vi "DataToVariant.vi"(1 "Data":string[][](table)) -> (0 "Variant":variant)   [LabVIEW 2014]
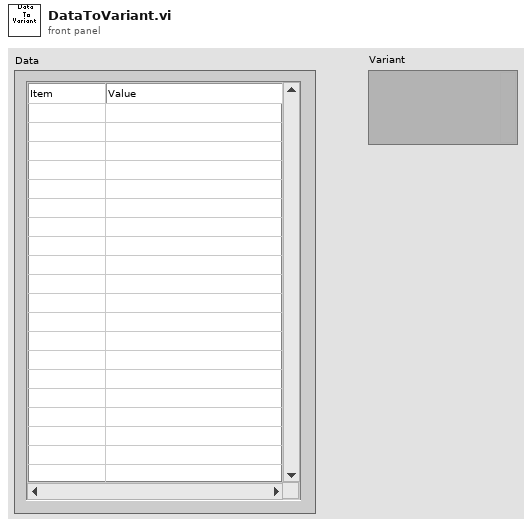
[diagram p1: front panel]
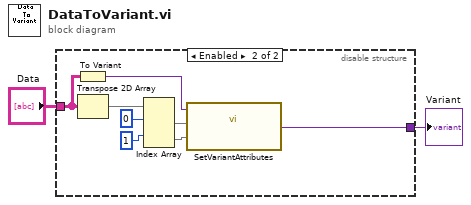
[diagram p0: block diagram]
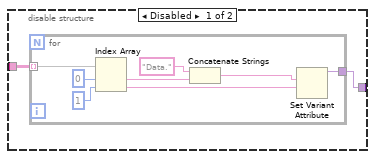
[diagram p2: hidden frame]
diagram:
  n1 = disable-structure shown="Enabled" {
    disable-tunnel: "Data" -> [w4 w20]
    disable-tunnel: [w3 w13] -> w1
    frame Disabled {
      n2 = for {
        tunnel: w4 -> [w12] mode=indexing
        tunnel: [w8] -> w3
        n3 = Index Array(array=w12, index #1=0 ("index"), index #2=1 ("index")) -> (element #1=w6:string, element #2=w9:string)
        n4 = Concatenate Strings("Data." ("string"), w6) -> (w5:string)
        n5 = Set Variant Attribute(name=w5, value=w9) -> (Variant out=w8:variant)  [unwired: 2 in, 2 out]
      }
    }
    frame Enabled {
      n6 = To Variant(anything=w20) -> (Variant=w14:variant)
      n7 = Transpose 2D Array(2D array=w20) -> (transposed array=w19:string[][])
      n8 = Index Array(array=w19, index (row) #1=0 ("index (row)"), index (row) #2=1 ("index (row)")) -> (element #1=w16:string[], element #2=w15:string[])  [unwired: 2 in]
      n9 = call "SetVariantAttributes.vi"("values"=w15, "names"=w16, "Variant In"=w14) -> ("Variant Out"=w13:variant)
    }
  }
  "Variant" <- w1
